vi "Test Spectrogram.vi"() -> ()   [LabVIEW 2020]
uses:
  Typedefs/ECOG-Parameters.ctl
  97e836ad-6d0f-47a7-a9a1-0932c3b6d51d.vi
  epl-vi-lib/Utility VIs/Math VIs/FFT x(t) to dB,Degrees (1D).vi
  <vilib>/Analysis/NI_AALBase.lvlib
panel:
  out "+Freq. Mag of FFT (dB rms)":dbl[](array[numeric])
  out "Intensity Graph":dbl[][](graph)
  in  "params":T1={"Channel"="", "Fs"=1000.0, "Frame Size"=100.0, "History Length"=5.0, "Filter"=FALSE, "Flo"=0.0, "Fhi"=0.0, "Fmax"=0.0, "Splitter Position"=0}
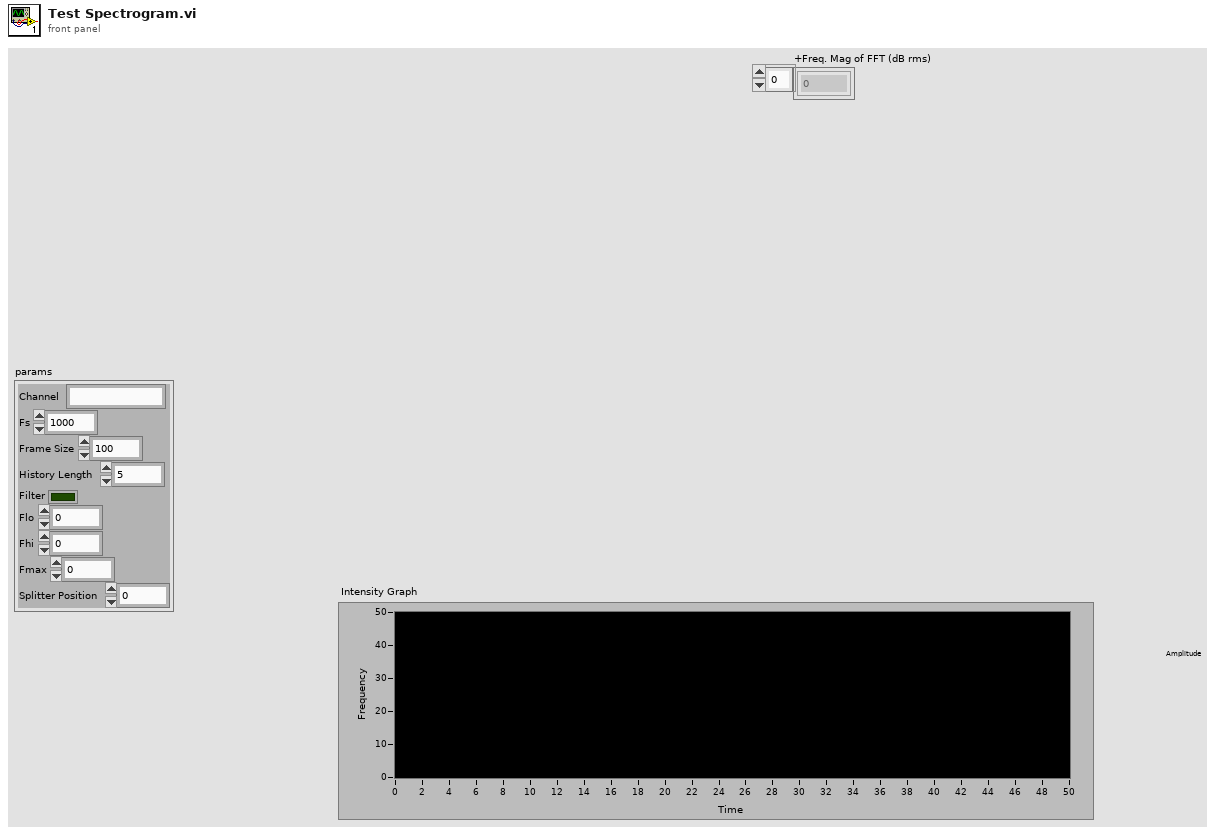
[diagram p1: front panel]
types:
  T1 = typedef "ECOG-Parameters.ctl" = cluster{"Channel":string, "Fs":dbl, "Frame Size":dbl, "History Length":dbl, "Filter":bool, "Flo":dbl, "Fhi":dbl, "Fmax":dbl, "Splitter Position":i32}
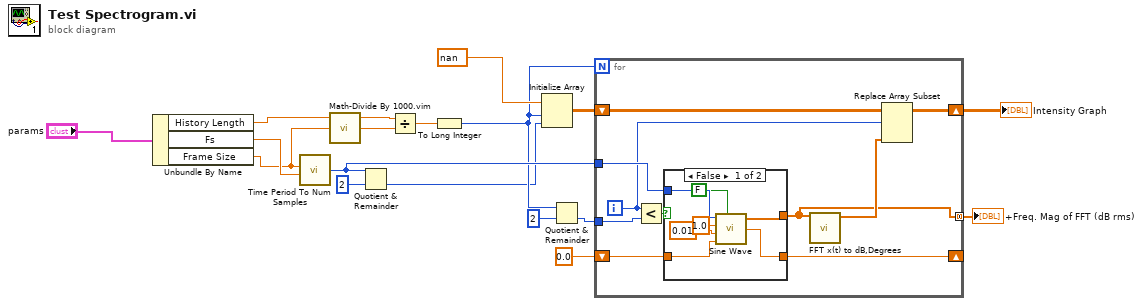
[diagram p0: block diagram]
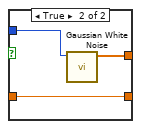
[diagram p2: hidden frame]
diagram:
  n1 = Unbundle By Name("params") -> ("History Length"=w15:dbl, "Fs"=w13:dbl, "Frame Size"=w11:dbl)
  n2 = call "Time Period To Num Samples.vi"("Duration (ms)"=w11, "Sampling rate (Hz)"=w13) -> ("Samples"=w6:i32)  [unwired: 5 in]
  n3 = call "Math-Divide By 1000.vim"("X"=w11) -> ("1000X"=w10:dbl)
  n4 = Quotient & Remainder(x=w6, y=2) -> (floor(x/y)=w1:i32)  [unwired: 1 out]
  n5 = Divide(x=w15, y=w10) -> (x/y=w14:dbl)
  n6 = To Long Integer(number=w14) -> (32bit integer=w2:i32)
  n7 = Initialize Array(nan, w2, w1) -> (w9:dbl[][])
  n8 = Quotient & Remainder(x=w2, y=2) -> (floor(x/y)=w7:i32)  [unwired: 1 out]
  n9 = for {
    N: w2 -> [_]
    shift-right: [w23] -> w5
    shift-left: w9 -> [w24]
    tunnel: w7 -> [w27]
    tunnel: w6 -> [w25]
    shift-right: [w21] -> _
    shift-left: 0.0 -> [w22]
    tunnel: [w19] -> w3 mode=concatenating
    i -> [w18]
    n10 = Less?(x=w18, y=w27) -> (x < y?=w26:bool)
    n11 = case shown="False" w26 {
      tunnel: w25 -> [w34 w37]
      tunnel: [w33 w36] -> w19
      tunnel: w22 -> [w32 w35]
      tunnel: [w31 w35] -> w21
      frame False {
        n12 = call <vilib>:"Sine Wave.vi"("samples"=w34, "amplitude"=1.0, "frequency"=0.01 ("amplitude"), "phase in"=w32, "reset phase"=FALSE) -> ("sine wave"=w33:dbl[], "phase out"=w31:dbl)  [unwired: 1 out]
      }
      frame True {
        n13 = call <vilib>:"Gaussian White Noise.vi"("samples"=w37) -> ("Gaussian noise pattern"=w36:dbl[])  [unwired: 9 in, 1 out]
      }
    }
    n14 = call-poly "FFT x(t) to dB,Degrees.vi"("X"=w19) -> ("+Freq. Mag of FFT (dB rms)"=w20:dbl[])  [unwired: 8 in, 2 out]
    n15 = Replace Array Subset(array=w24, new element=w20, index (row)=w18) -> (w23:dbl[][])  [unwired: 1 in]
  }
  "Intensity Graph" <- w5
  "+Freq. Mag of FFT (dB rms)" <- w3
